vi "PlotCylparams.vi"() -> ()   [LabVIEW 2014]
uses:
  TypeDefs/RectHatch.ctl
  TypeDefs/PowerSpeed.ctl
  <vilib>/Utility/file.llb/Read From Spreadsheet File (DBL).vi
panel:
  out "Params":cluster{dbl, dbl, dbl, dbl, dbl}[](array[cluster])
  in  "CircHatch":T1={"Diameter"=1.6, "Angle"=45.0, "Offset"=0.05, "Spacing"=0.1} {"Spacing" format="%#_13g"; "Offset" format="%#_13g"; "Diameter" format="%#_13g"}
  in  "DummyCubeLoc":cluster{dbl, dbl}={-30.0, 30.0}
  in  "Save?":bool=TRUE
  in  "Path":path=path "\\\\nif-prgms-srvr.llnl.gov\\LMOT/Damage Group/Matthews/AM/fraunhofer SLM/BuildFiles_STL_ILT/SCN/DogBoneAndCylinders_11-23-16"
  in  "HighPower":dbl=300.0
  in  "Display":T2={"Mode"=enum."Inherit Value", "PointSize"=1.0, "LineWidth"=1.0}
  in  "LayerEnd":u32=266
  in  "LayerStart":u32
  in  "HatchPow":T3={"Power"=350.0, "Mark Speed"=300.0, "Jump Speed"=1000.0, "JumpPower"=0.0}
  in  "RectHatch":T4={"Width"=10.0, "Height"=1.0, "Angle"=45.0, "OffX"=0.1, "OffY"=0.1, "Spacing"=0.1, "IslandSize"=0.1} {"IslandSize" format="%#_13g"; "Spacing" format="%#_13g"; "OffY" format="%#_13g"; "OffX" format="%#_13g"; "Height" format="%#_13g"; "Width" format="%#_13g"}
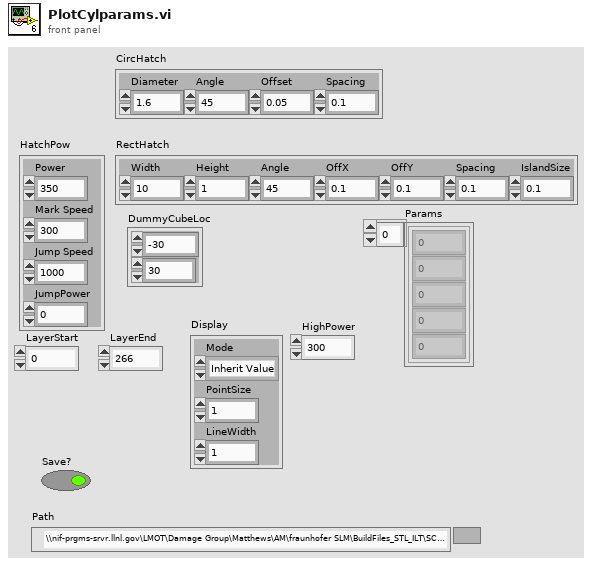
[diagram p1: front panel]
types:
  T1 = cluster{"Diameter":dbl, "Angle":sgl, "Offset":dbl, "Spacing":dbl}
  T2 = cluster{"Mode":enum16{"Inherit Value", "Points", "Wireframe", "Polygons"}, "PointSize":sgl, "LineWidth":sgl}
  T3 = typedef "PowerSpeed.ctl" = cluster{"Power":dbl, "Mark Speed":dbl, "Jump Speed":dbl, "JumpPower":dbl}
  T4 = typedef "RectHatch.ctl" = cluster{"Width":dbl, "Height":dbl, "Angle":sgl, "OffX":dbl, "OffY":dbl, "Spacing":dbl, "IslandSize":dbl}
  T5 = typedef "PathSupreme.ctl" = cluster{"VelocityProfiles":T6[], "Path":T7}
  T6 = typedef "VelocityProfile.ctl" = cluster{"ID":u32, "Velocity":dbl, "Mode":string, "tV1":u32, "tV2":u32, "tL1":u32, "tL2":u32}
  T7 = typedef "PathCut.ctl" = cluster{"Type":string, "Tag":string, "Segments":T8[]}
  T8 = typedef "Segment.ctl" = cluster{"SegmentID":u16, "Power":sgl, "idxVelocityProfile":u16, "End":cluster{"X":sgl, "Y":sgl}}
  T9 = typedef "Point3D.ctl" = cluster{"X":sgl, "Y":sgl, "Z":sgl}
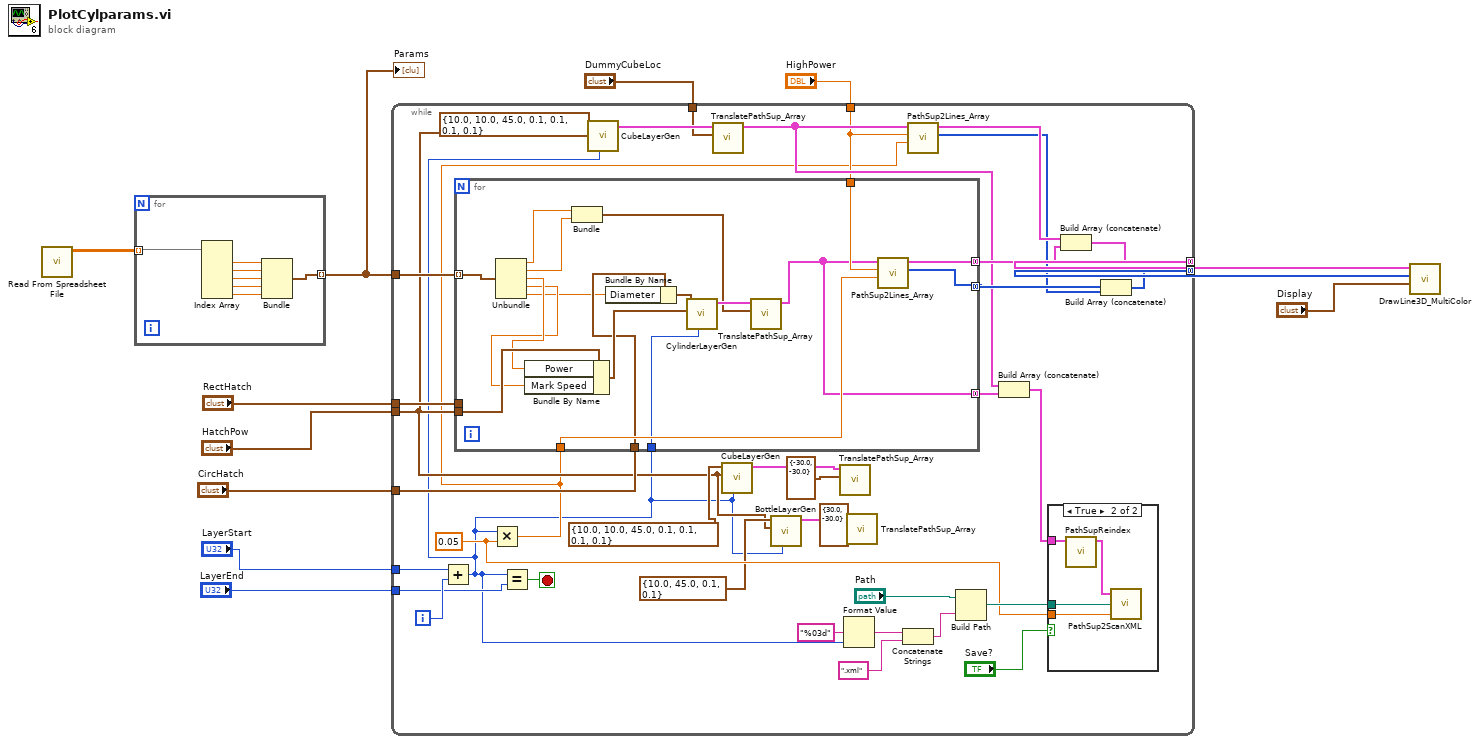
[diagram p0: block diagram]
diagram:
  n1 = call-poly <vilib>:"Read From Spreadsheet File.vi"() -> ("all rows"=w12:dbl[][])  [unwired: 7 in, 4 out]
  n2 = for {
    tunnel: w12 -> [w19] mode=indexing
    tunnel: [w14] -> w7 mode=indexing
    n3 = Index Array(array=w19) -> (element #1=w17:dbl, element #2=w18:dbl, element #3=w16:dbl, element #4=w15:dbl, element #5=w13:dbl)  [unwired: 5 in]
    n4 = Bundle(w17, w18, w16, w15, w13) -> (w14:cluster{dbl, dbl, dbl, dbl, dbl})  [unwired: 1 in]
  }
  "Params" <- w7
  n5 = while {
    tunnel: "HighPower" -> [w22]
    tunnel: [w39] -> w10 mode=concatenating
    tunnel: [w36] -> w9 mode=concatenating
    tunnel: w7 -> [w54]
    tunnel: "RectHatch" -> [w32]
    tunnel: "HatchPow" -> [w25]
    tunnel: "LayerEnd" -> [w53]
    tunnel: "LayerStart" -> [w52]
    tunnel: "DummyCubeLoc" -> [w42]
    tunnel: "CircHatch" -> [w31]
    i -> [w56]
    stop <- w55 stop-if-true
    w45 = 0.05 ("y")
    n6 = Add(x=w52, y=w56) -> (x+y=w20:u32)
    n7 = Multiply(x=w20, y=w45) -> (x*y=w21:dbl)
    n8 = for {
      tunnel: w20 -> [w69]
      tunnel: w21 -> [w76]
      tunnel: w22 -> [w75]
      tunnel: [w78] -> w40 mode=concatenating
      tunnel: w54 -> [w77] mode=indexing
      tunnel: w32 -> [_]
      tunnel: w25 -> [w73]
      tunnel: [w65] -> w35 mode=concatenating
      tunnel: [w74] -> w38 mode=concatenating
      tunnel: w31 -> [w63]
      n9 = Unbundle(w77) -> (w64:dbl, w68:dbl, w72:dbl, w71:dbl, w61:dbl)
      n10 = Bundle By Name(cluster=w73, "Power"=w72, "Mark Speed"=w71) -> (w70:T3)
      n11 = Bundle(w64, w68) -> (w66:cluster{dbl, dbl})  [unwired: 1 in]
      n12 = Bundle By Name(cluster=w63, "Diameter"=w61) -> (w62:T1)
      n13 = call "CylinderLayerGen.vi"("Layer"=w69, "HatchPow"=w70, "CircHatch"=w62) -> ("PathSups"=w67:T5[])  [unwired: 8 in]
      n14 = call "TranslatePathSup_Array.vi"("Offset"=w66, "PathSupsIn"=w67) -> ("PathSupsOut"=w65:T5[])  [unwired: 9 in]
      n15 = call "PathSup2Lines_Array.vi"("Z"=w76, "HighPower"=w75, "PathSupIn"=w65) -> ("Colors"=w74:u32[], "Lines"=w78:cluster{"P0":T9, "P1":T9}[])  [unwired: 7 in]
    }
    n16 = Equal?(x=w20, y=w53) -> (x = y?=w55:bool)
    n17 = call "CubeLayerGen.vi"("Layer"=w20, "HatchPow"=w25, "RectHatch"=T4 {"Width"=10.0, "Height"=10.0, "Angle"=45.0, "OffX"=0.1, "OffY"=0.1, "Spacing"=0.1, "IslandSize"=0.1}) -> ("PathSups"=w43:T5[])  [unwired: 8 in]
    n18 = call "TranslatePathSup_Array.vi"("Offset"=w42, "PathSupsIn"=w43) -> ("PathSupsOut"=w34:T5[])  [unwired: 9 in]
    n19 = call "CubeLayerGen.vi"("Layer"=w20, "HatchPow"=w25, "RectHatch"=T4 {"Width"=10.0, "Height"=10.0, "Angle"=45.0, "OffX"=0.1, "OffY"=0.1, "Spacing"=0.1, "IslandSize"=0.1}) -> ("PathSups"=w28:T5[])  [unwired: 8 in]
    n20 = call "BottleLayerGen.vi"("Layer"=w20, "HatchPow"=w25, "CircHatch"=T1 {"Diameter"=10.0, "Angle"=45.0, "Offset"=0.1, "Spacing"=0.1}) -> ("PathSups"=w24:T5[])  [unwired: 8 in]
    n21 = call "TranslatePathSup_Array.vi"("Offset"=cluster{dbl, dbl} {-30.0, -30.0}, "PathSupsIn"=w28) -> ()  [unwired: 9 in, 1 out]
    n22 = Format Value(format string="%03d", value (0)=w20) -> (output string=w50:string)  [unwired: 1 in]
    n23 = call "TranslatePathSup_Array.vi"("Offset"=cluster{dbl, dbl} {30.0, -30.0}, "PathSupsIn"=w24) -> ()  [unwired: 9 in, 1 out]
    n24 = Concatenate Strings(w50, ".xml" ("string")) -> (w48:string)
    n25 = call "PathSup2Lines_Array.vi"("Z"=w21, "HighPower"=w22, "PathSupIn"=w34) -> ("Colors"=w37:u32[], "Lines"=w41:cluster{"P0":T9, "P1":T9}[])  [unwired: 7 in]
    n26 = Build Path(base path="Path", name or relative path=w48) -> (appended path=w46:path)
    n27 = Build Array (concatenate)(w34, w35) -> (w33:T5[])
    n28 = case shown="True" "Save?" {
      tunnel: w33 -> [_ w58]
      tunnel: w46 -> [_ w60]
      tunnel: w45 -> [_ w59]
      frame False {
      }
      frame True {
        n29 = call "PathSupReindex.vi"("PathSupremes"=w58) -> ("PathSupOut"=w57:T5[])  [unwired: 10 in]
        n30 = call "PathSup2ScanXML.vi"("Thickness"=w59, "Path"=w60, "PathSupremes"=w57) -> ()  [unwired: 2 in, 1 out]
      }
    }
    n31 = Build Array (concatenate)(w41, w40) -> (w39:cluster{"P0":T9, "P1":T9}[])
    n32 = Build Array (concatenate)(w38, w37) -> (w36:u32[])
  }
  n33 = call "DrawLine3D_MultiColor.vi"("Display"="Display", "Colors"=w9, "Lines"=w10) -> ()  [unwired: 9 in]
